vi "T2_KeyToValue.vi"(4 "Keys":cluster{"Start":u64, "End":u64}[](array[cluster]), 5 "String":string) -> (0 "Source > Dest":T1(c390), 1 "Values":cluster{"Start":u64, "End":u64}[](array[cluster]))   [LabVIEW 2022 SP3]
panel:
  out "Array":u32[](array[numeric])
  out "appended array":bool[][](array[boolean])
  out "Array 2":cluster{"Start":u64, "End":u64}[][](array[cluster])
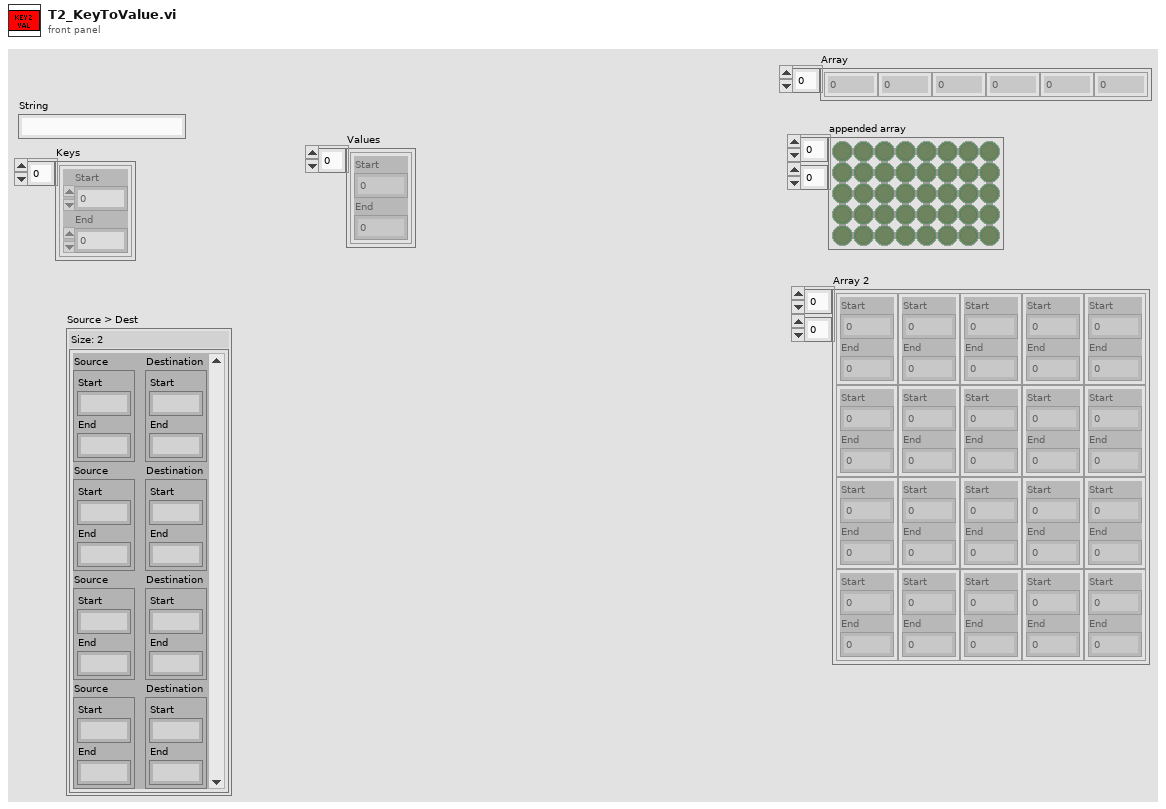
[diagram p1: front panel]
types:
  T1 = map{cluster{"Start":u64, "End":u64}, cluster{"Start":u64, "End":u64}}
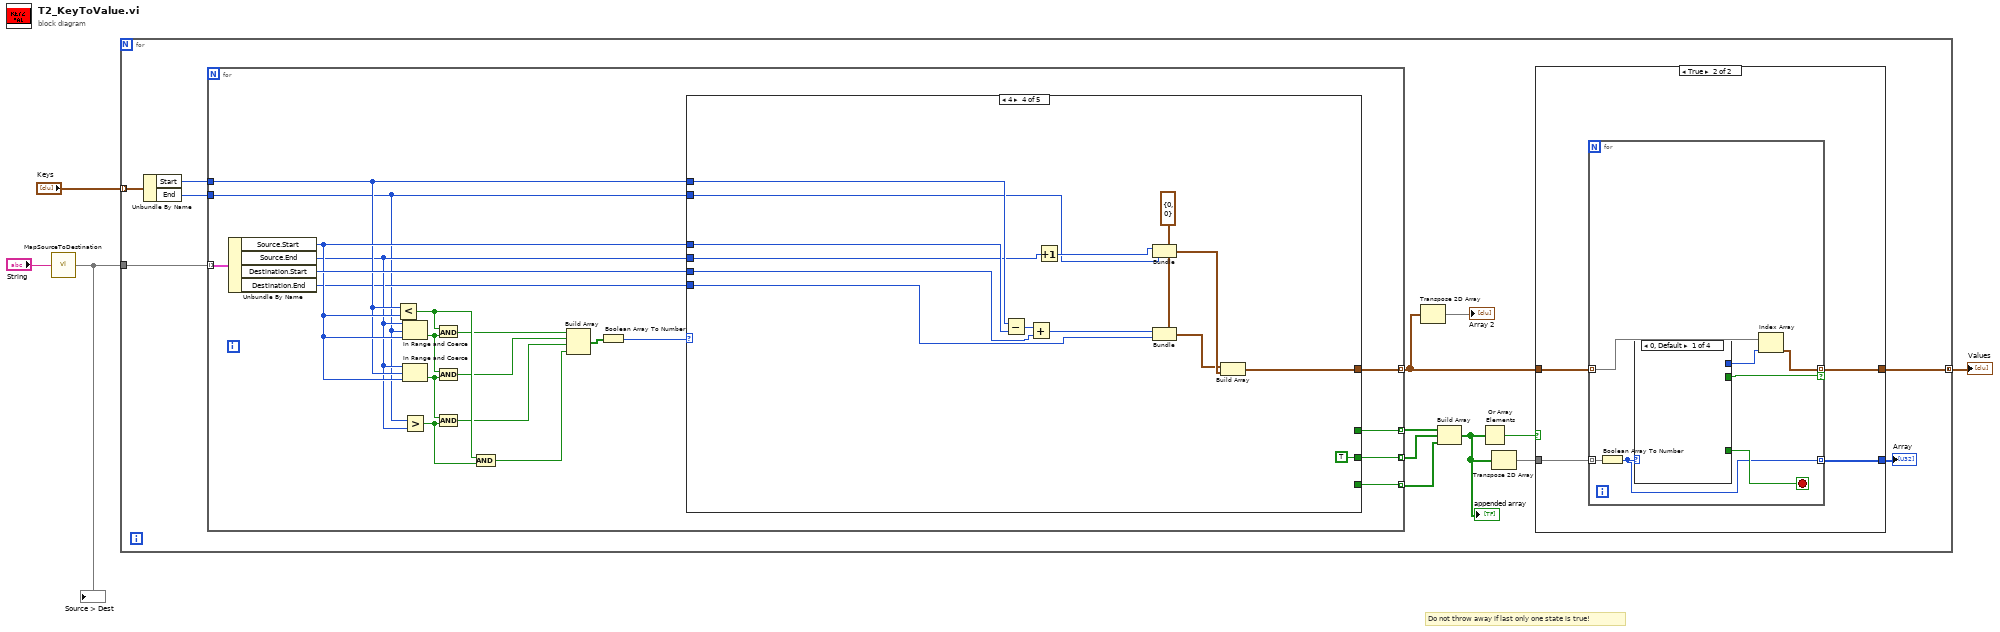
[diagram p0: block diagram]
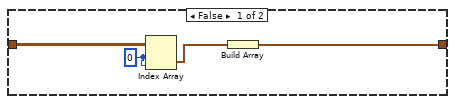
[diagram p2: hidden frame]
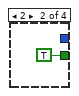
[diagram p3: hidden frame]
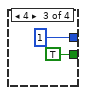
[diagram p4: hidden frame]
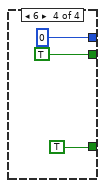
[diagram p5: hidden frame]
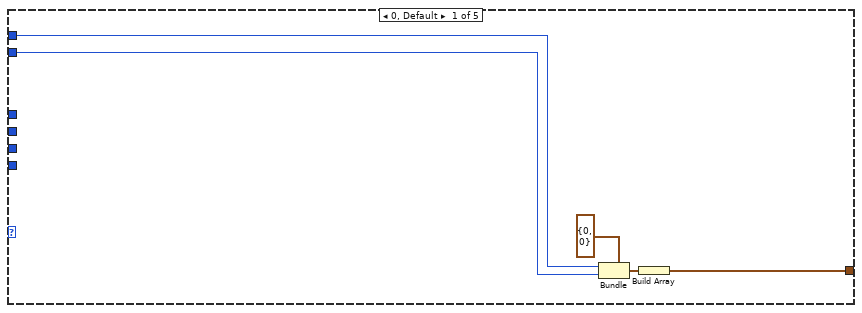
[diagram p6: hidden frame]
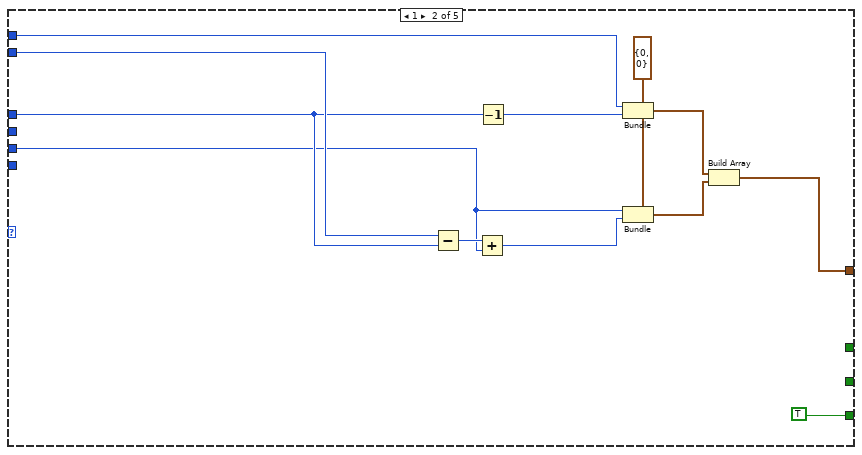
[diagram p7: hidden frame]
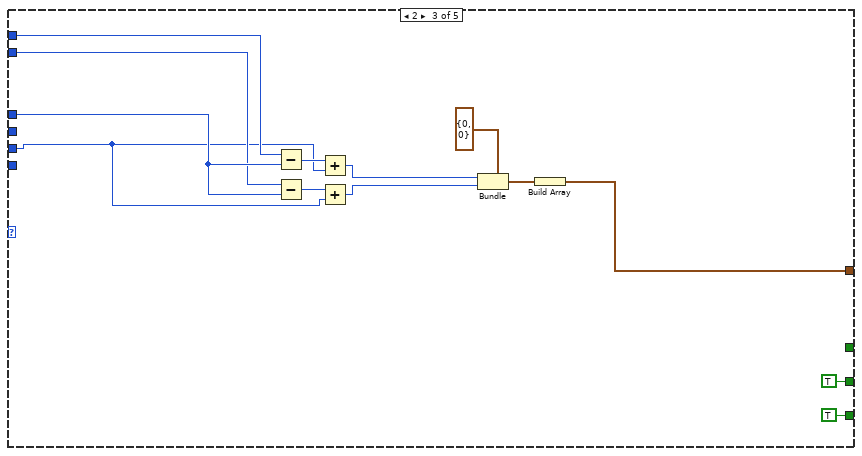
[diagram p8: hidden frame]
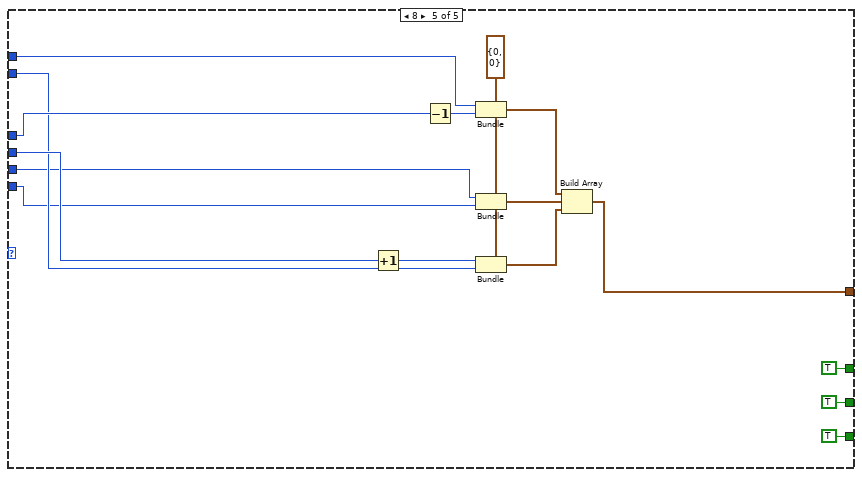
[diagram p9: hidden frame]
diagram:
  # "Do not throw away if last only one state is true!"
  n1 = call "MapSourceToDestination.vi"("String"="String") -> ("Source > Dest"=w3:T1)  [unwired: 6 in]
  "Source > Dest" <- w3
  n2 = for {
    tunnel: "Keys" -> [w18] mode=indexing
    tunnel: w3 -> [w16]
    tunnel: [w8] -> w1 mode=concatenating
    n3 = Unbundle By Name(w18) -> ("Start"=w17:u64, "End"=w15:u64)
    n4 = for {
      tunnel: w16 -> [w60] mode=indexing
      tunnel: w17 -> [w57]
      tunnel: w15 -> [w44]
      tunnel: [w43] -> w9 mode=indexing
      tunnel: [w42] -> w13 mode=indexing
      tunnel: [w41] -> w12 mode=indexing
      tunnel: [w40] -> w14 mode=indexing
      n5 = Unbundle By Name(w60) -> ("Source.Start"=w58:u64, "Source.End"=w55:u64, "Destination.Start"=w59:u64, "Destination.End"=w45:u64)
      n6 = Less?(x=w57, y=w58) -> (x < y?=w53:bool)
      n7 = In Range and Coerce(upper limit=w55, x=w44, lower limit=w58) -> (In Range?=w56:bool)  [unwired: 1 out]
      n8 = In Range and Coerce(upper limit=w55, x=w57, lower limit=w58) -> (In Range?=w54:bool)  [unwired: 1 out]
      n9 = Greater?(x=w44, y=w55) -> (0:w52:bool)
      n10 = And(x=w53, y=w56) -> (x .and. y?=w51:bool)
      n11 = And(x=w56, y=w54) -> (x .and. y?=w50:bool)
      n12 = And(x=w54, y=w52) -> (x .and. y?=w49:bool)
      n13 = And(x=w53, y=w52) -> (x .and. y?=w48:bool)
      n14 = Build Array(w51, w50, w49, w48) -> (w47:bool[])
      n15 = Boolean Array To Number(Boolean array=w47) -> (number=w46:u32)
      n16 = case shown="4" w46 {
        tunnel: [w63 w77 w80 w92 w108] -> w43
        tunnel: w44 -> [w62 w69 w82 w93 w111]
        tunnel: w57 -> [w61 w70 w84 w100 w114]
        tunnel: w58 -> [_ w68 w83 w99 w113]
        tunnel: w55 -> [_ _ _ w95 w112]
        tunnel: w59 -> [_ w67 w81 w97 w110]
        tunnel: w45 -> [_ _ _ w96 w109]
        tunnel: [_ _ TRUE TRUE TRUE] -> w42
        tunnel: [_ TRUE TRUE _ TRUE] -> w41
        tunnel: [_ _ _ _ TRUE] -> w40
        frame 0, Default {
          n17 = Bundle(cluster=cluster{"Start":u64, "End":u64} {"Start"=0, "End"=0} ("Source"), "Start"=w61, "End"=w62) -> (w64:cluster{"Start":u64, "End":u64})
          n18 = Build Array(w64) -> (w63:cluster{"Start":u64, "End":u64}[])
        }
        frame 1 {
          w76 = cluster{"Start":u64, "End":u64} {"Start"=0, "End"=0} ("Source")
          n19 = Subtract(x=w69, y=w68) -> (x-y=w72:u64)
          n20 = Add(x=w72, y=w67) -> (x+y=w71:u64)
          n21 = Decrement(x=w68) -> (x-1=w75:u64)
          n22 = Bundle(cluster=w76, "Start"=w70, "End"=w75) -> (w74:cluster{"Start":u64, "End":u64})
          n23 = Bundle(cluster=w76, "Start"=w67, "End"=w71) -> (w73:cluster{"Start":u64, "End":u64})
          n24 = Build Array(w74, w73) -> (w77:cluster{"Start":u64, "End":u64}[])
        }
        frame 2 {
          n25 = Subtract(x=w84, y=w83) -> (x-y=w88:u64)
          n26 = Subtract(x=w82, y=w83) -> (x-y=w87:u64)
          n27 = Add(x=w88, y=w81) -> (x+y=w86:u64)
          n28 = Add(x=w87, y=w81) -> (x+y=w85:u64)
          n29 = Bundle(cluster=cluster{"Start":u64, "End":u64} {"Start"=0, "End"=0} ("Source"), "Start"=w86, "End"=w85) -> (w89:cluster{"Start":u64, "End":u64})
          n30 = Build Array(w89) -> (w80:cluster{"Start":u64, "End":u64}[])
        }
        frame 4 {
          w104 = cluster{"Start":u64, "End":u64} {"Start"=0, "End"=0} ("Source")
          n31 = Subtract(x=w100, y=w99) -> (x-y=w101:u64)
          n32 = Add(x=w101, y=w97) -> (x+y=w98:u64)
          n33 = Increment(x=w95) -> (x+1=w94:u64)
          n34 = Bundle(cluster=w104, "Start"=w94, "End"=w93) -> (w103:cluster{"Start":u64, "End":u64})
          n35 = Bundle(cluster=w104, "Start"=w98, "End"=w96) -> (w102:cluster{"Start":u64, "End":u64})
          n36 = Build Array(w102, w103) -> (w92:cluster{"Start":u64, "End":u64}[])
        }
        frame 8 {
          w117 = cluster{"Start":u64, "End":u64} {"Start"=0, "End"=0} ("Source")
          n37 = Increment(x=w112) -> (x+1=w115:u64)
          n38 = Decrement(x=w113) -> (x-1=w116:u64)
          n39 = Bundle(cluster=w117, "Start"=w114, "End"=w116) -> (w120:cluster{"Start":u64, "End":u64})
          n40 = Bundle(cluster=w117, "Start"=w110, "End"=w109) -> (w119:cluster{"Start":u64, "End":u64})
          n41 = Bundle(cluster=w117, "Start"=w115, "End"=w111) -> (w118:cluster{"Start":u64, "End":u64})
          n42 = Build Array(w120, w119, w118) -> (w108:cluster{"Start":u64, "End":u64}[])
        }
      }
    }
    n43 = Transpose 2D Array(2D array=w9) -> (transposed array=→"Array 2":cluster{"Start":u64, "End":u64}[][])
    n44 = Build Array(w14, w13, w12) -> (w7:bool[][])
    "appended array" <- w7
    n45 = Or Array Elements(Boolean array=w7) -> (logical OR=w10:bool)
    n46 = Transpose 2D Array(2D array=w7) -> (transposed array=w5:bool[][])
    n47 = case shown="True" w10 {
      tunnel: w9 -> [w22 w25]
      tunnel: [w19 w23] -> w8
      tunnel: w5 -> [_ w26]
      tunnel: [_ w24] -> w6
      frame False {
        w21 = 0 ("index (row)")
        n48 = Index Array(array=w22, index (row)=w21, index (col)=w21) -> (element=w20:cluster{"Start":u64, "End":u64})
        n49 = Build Array(w20) -> (w19:cluster{"Start":u64, "End":u64}[])
      }
      frame True {
        n50 = for {
          tunnel: w26 -> [w33] mode=indexing
          tunnel: w25 -> [w27] mode=indexing
          tunnel: [w29] -> w23 mode=indexing if=w30
          tunnel: [w31] -> w24 mode=indexing
          stop <- w32 stop-if-true
          n51 = Boolean Array To Number(Boolean array=w33) -> (number=w31:u32)
          n52 = case shown="0, Default" w31 {
            tunnel: [_ _ _ TRUE] -> w32
            tunnel: [_ TRUE TRUE TRUE] -> w30
            tunnel: [_ _ 1 0 ("index")] -> w28
            frame 0, Default {
            }
            frame 2 {
            }
            frame 4 {
            }
            frame 6 {
            }
          }
          n53 = Index Array(array=w27, index=w28) -> (element=w29:cluster{"Start":u64, "End":u64})
        }
      }
    }
    "Array" <- w6
  }
  "Values" <- w1
